vi "demo.vi"() -> ()   [LabVIEW 2018]
uses:
  sheep/Sheep.lvclass
  tiger/Tiger.lvclass
  cow/Cow.lvclass
  animal/Animal.lvclass
panel:
  out "Array":string[](array[string])
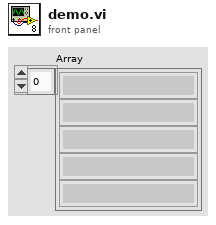
[diagram p1: front panel]
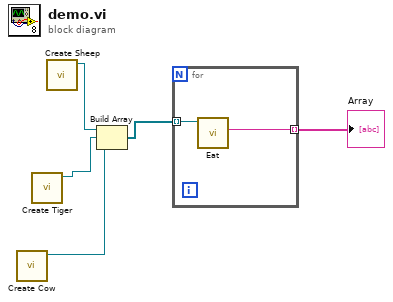
[diagram p0: block diagram]
diagram:
  n1 = call "Create Cow.vi"() -> ("Cow.lvclass"=w1:refnum<class "Cow.lvclass">)  [unwired: 11 in]
  n2 = call "Create Tiger.vi"() -> ("output cluster"=w4:refnum<class "Tiger.lvclass">)  [unwired: 11 in]
  n3 = call "Create Sheep.vi"() -> ("Sheep.lvclass"=w5:refnum<class "Sheep.lvclass">)  [unwired: 11 in]
  n4 = Build Array(w5, w4, w1) -> (w3:refnum<class "Animal.lvclass">[])
  n5 = for {
    tunnel: w3 -> [w7] mode=indexing
    tunnel: [w6] -> w2 mode=indexing
    n6 = call-dynamic "Eat.vi"("Animal in"=w7) -> ("String 2"=w6:string)  [unwired: 8 in, 2 out]
  }
  "Array" <- w2
